vi "test_angle bugcheck.vi"() -> ()   [LabVIEW 2019]
panel:
  out "deg_gps-base 2":dbl=99.99122768605022 format="%.1f"
  in  "agv curr utm out":cluster{dbl, dbl}={175444.42435705324, 530246.6811099245} {"?" format="%.2f"; "?" format="%.2f"}
  in  "lookahead-1 9164":cluster{"x":dbl, "y":dbl}={"x"=175442.57659798823, "y"=530247.4558224457} {"x" format="%.2f"; "y" format="%.2f"}
  out "deg_gps-base":dbl=99.9978218841811 format="%.1f"
  in  "agv curr utm 9163":cluster{dbl, dbl}={175444.40035197235, 530246.6836853756} {"?" format="%.2f"; "?" format="%.2f"}
  in  "lookahead-1 9163":cluster{"x":dbl, "y":dbl}={"x"=175446.3907214257, "y"=530246.783357573} {"x" format="%.2f"; "y" format="%.2f"}
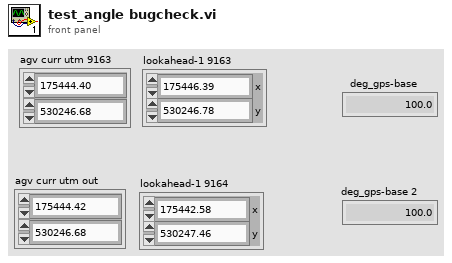
[diagram p1: front panel]
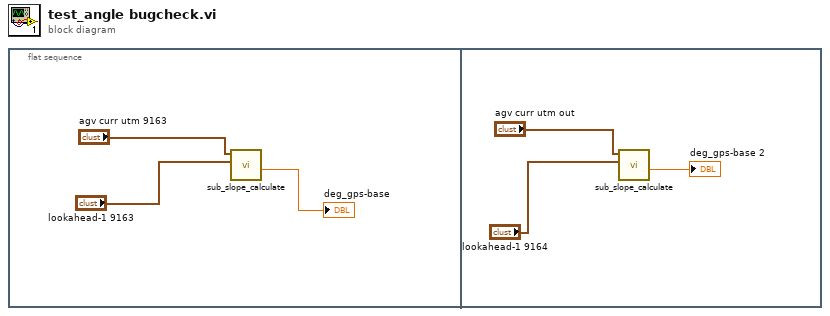
[diagram p0: block diagram]
diagram:
  n1 = flat-sequence {
    frame #0 {
      n2 = call "sub_slope_calculate.vi"("point n+1"="lookahead-1 9163", "point n"="agv curr utm 9163") -> ("deg_gps-base"=→"deg_gps-base":dbl)  [unwired: 7 in, 2 out]
    }
    frame #1 {
      n3 = call "sub_slope_calculate.vi"("point n+1"="lookahead-1 9164", "point n"="agv curr utm out") -> ("deg_gps-base"=→"deg_gps-base 2":dbl)  [unwired: 7 in, 2 out]
    }
  }
